vi "Day01-01.vi"() -> ()   [LabVIEW 2021]
panel:
  out "삭제된 부분":dbl[](array[numeric])
  out "부분이 삭제된 배열":dbl[](array[numeric])
  out "출력 배열":dbl[](array[numeric])
  out "원소 3":dbl
  out "원소 2":dbl
  out "원소":dbl
  out "크기 2":i32[](array[numeric])
  out "크기":i32
  in  "2D 배열":dbl[][](array[numeric])
  in  "1D 배열":dbl[](array[numeric])
  in  "배열":dbl[](array[numeric])
  in  "2차원 배열":dbl[][](array[numeric])
  in  "1차원 배열 2":dbl[](array[numeric])
  in  "1차원 배열":dbl[](array[numeric])
  in  "숫자형 11":dbl
  out "0, 1":i16
  out "결과 문자열 2":string
  out "결과 문자열":string
  out "숫자 2":i32
  out "10진수 문자열":string
  out "숫자":i32
  in  "문자열 8":string
  out "문자열 7":string
  in  "문자열 6":string
  in  "문자열 5":string
  in  "문자열 4":string
  out "길이":i32
  in  "문자열 3":string
  in  "불리언 3":bool
  out "숫자형 10":dbl
  out "32비트 정수":i32
  in  "숫자형 9":i32
  in  "숫자형 8":dbl
  in  "숫자형 7":dbl
  out "X + Y":dbl
  in  "숫자형 5":u8
  in  "숫자형 4":u8
  out "가장 가까운 정수값":dbl
  in  "숫자형 3":u32
  out "숫자형 6":dbl
  in  "Y":dbl
  in  "X":dbl
  out "불리언 2":bool
  in  "불리언":bool
  out "문자열 2":string
  in  "문자열":string
  out "숫자형 2":dbl
  in  "숫자형":dbl
  # "배열"
  # "예제 4-1"
  # "예제 4-4"
  # "원소"
  # "인덱스"
  # "예제 4-2"
  # "예제 4-5"
  # "예제 4-3"
  # "원소의 개수는? \n --> 5개"
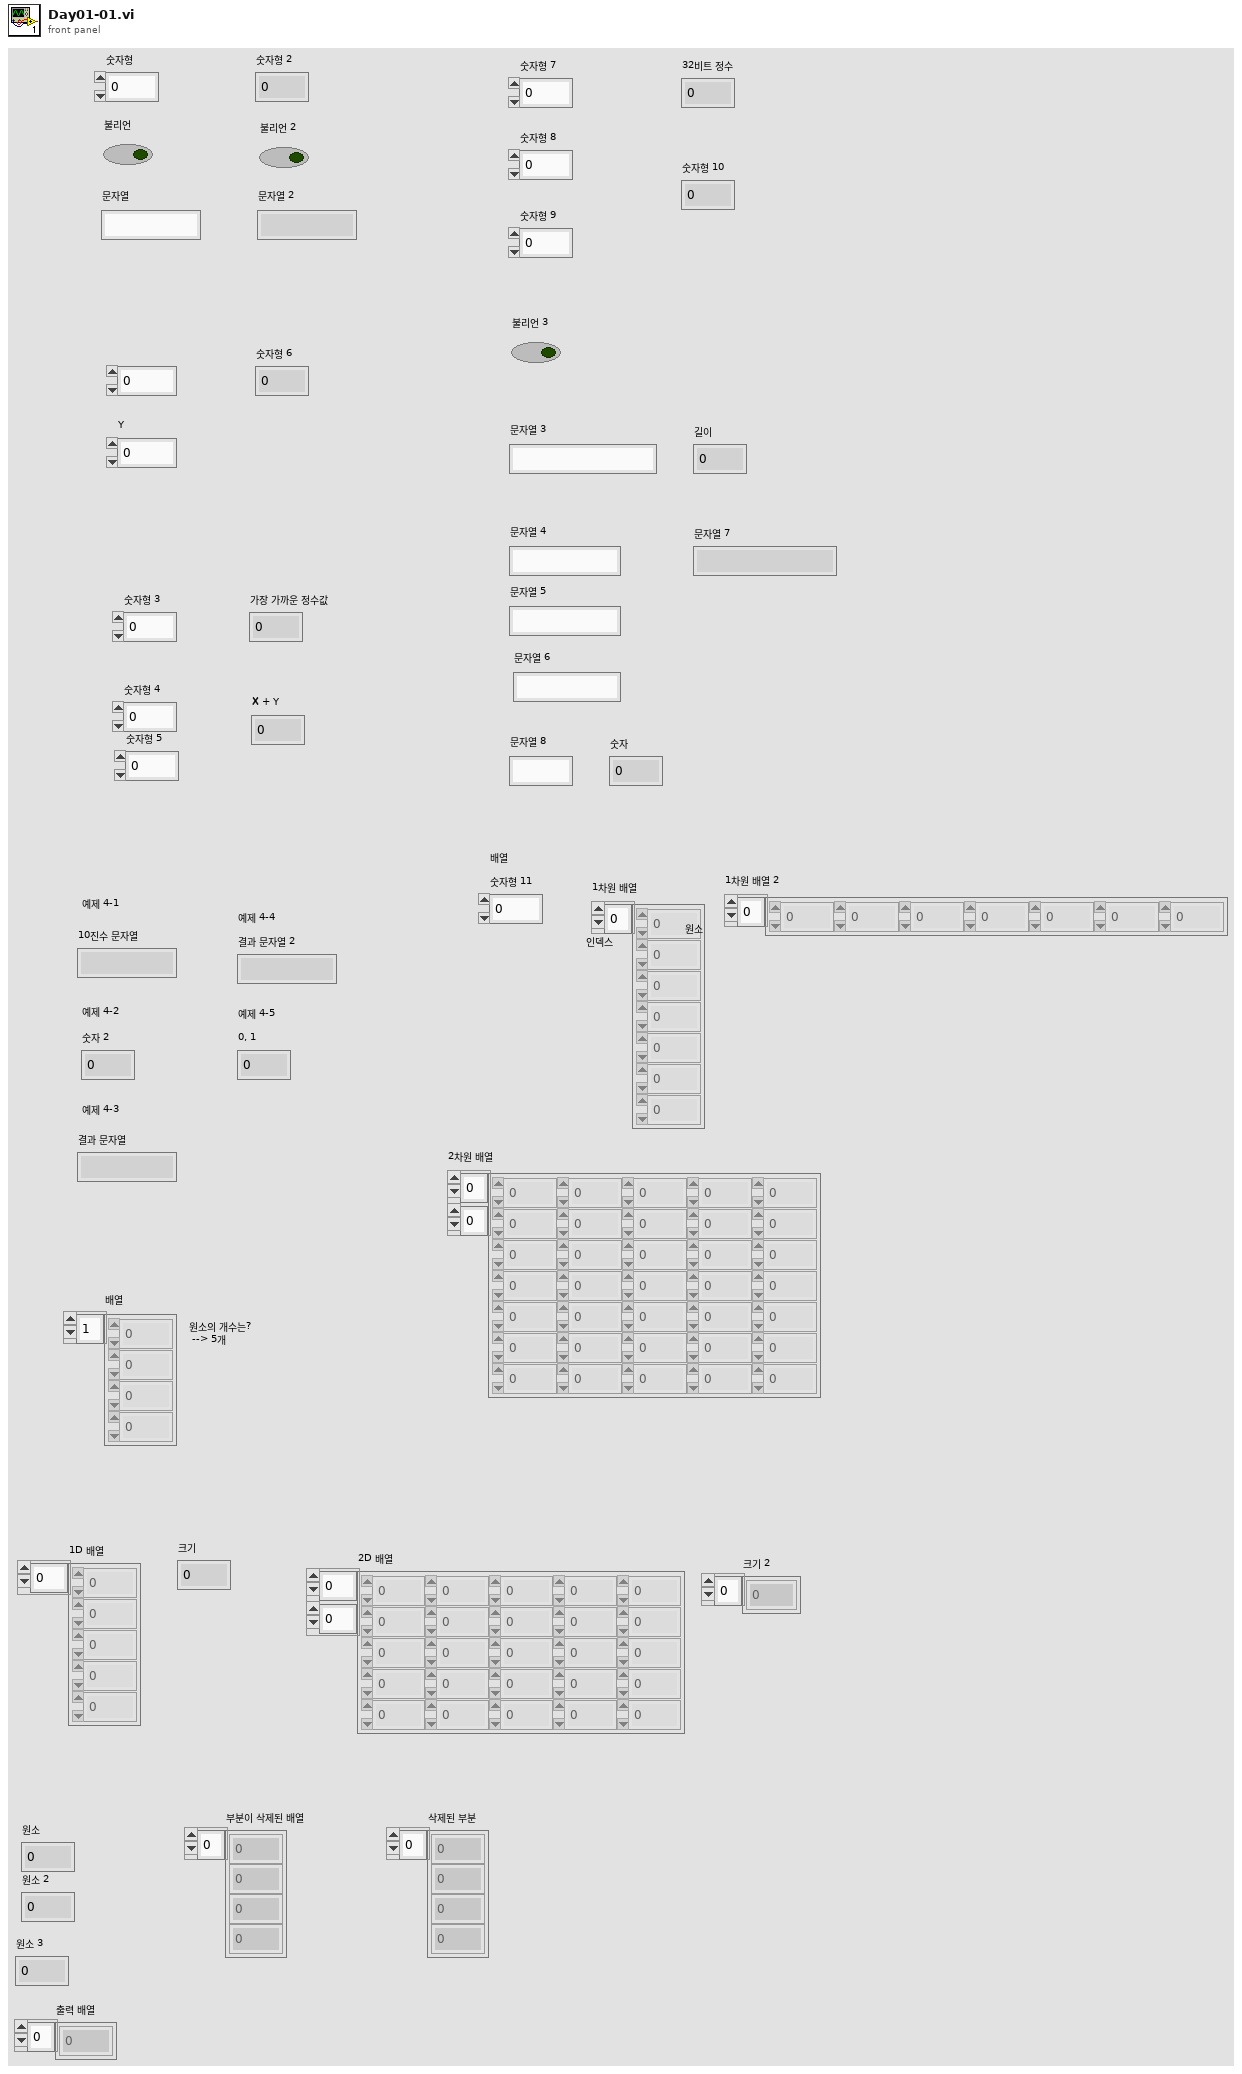
[diagram p1: front panel]
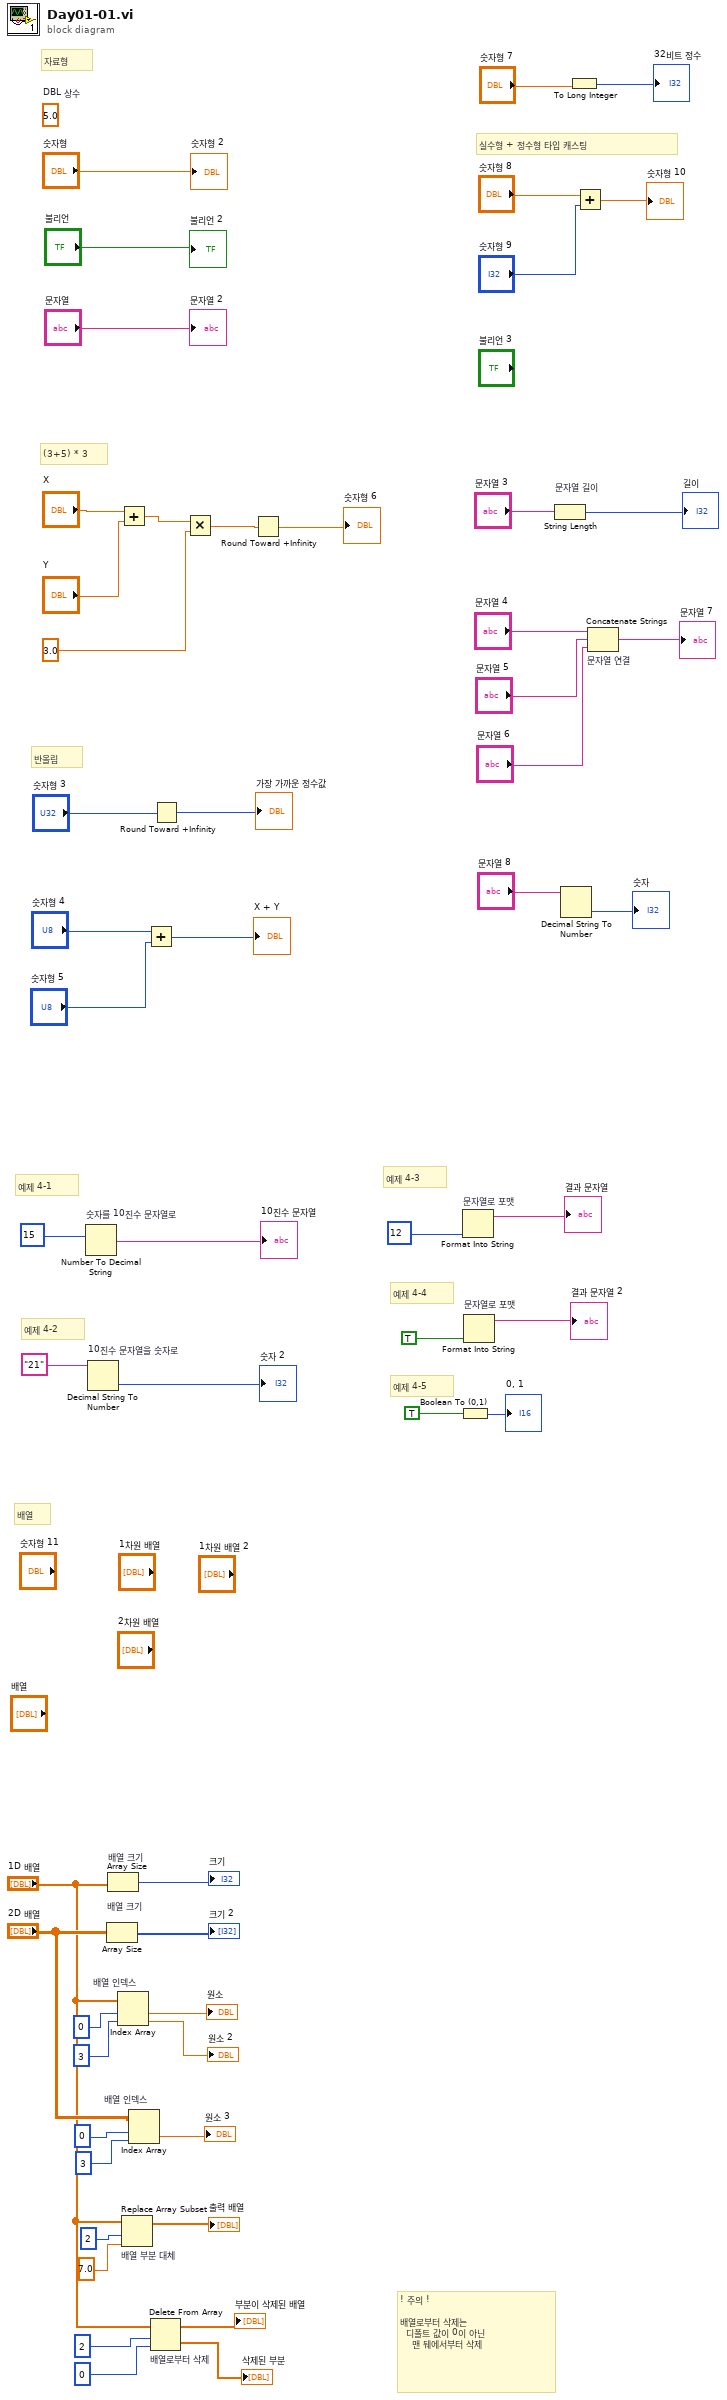
[diagram p0: block diagram]
diagram:
  (unwired) 5.0  # DBL 상수
  # "! 주의 !\n\n배열로부터 삭제는\n  디폴트 값이 0이 아닌\n    맨 뒈에서부터 삭제"
  # "배열"
  # "예제 4-5"
  # "예제 4-4"
  # "예제 4-3"
  # "예제 4-2"
  # "예제 4-1"
  # "실수형 + 정수형 타입 캐스팅"
  # "반올림"
  # "(3+5) * 3"
  # "자료형"
  n1 = Number To Decimal String "숫자를 10진수 문자열로"(number=15) -> (decimal integer string=→"10진수 문자열":string)  [unwired: 1 in]
  n2 = Decimal String To Number "10진수 문자열을 숫자로"(string="21") -> (number=→"숫자 2":i32)  [unwired: 2 in, 1 out]
  n3 = Array Size "배열 크기"(array="2D 배열") -> (size(s)=→"크기 2":i32[])
  n4 = Array Size "배열 크기"(array="1D 배열") -> (size(s)=→"크기":i32)
  n5 = Index Array "배열 인덱스"(array="1D 배열", index #1=0, index #2=3) -> (element #1=→"원소":dbl, element #2=→"원소 2":dbl)
  n6 = Add(x="X", y="Y") -> (x+y=w50:dbl)
  n7 = Replace Array Subset "배열 부분 대체"(array="1D 배열", new element=7.0 ("새 원소/부분배열"), index=2 ("인덱스")) -> (→"출력 배열":dbl[])
  n8 = Index Array "배열 인덱스"(array="2D 배열", index (row)=0, index (col)=3) -> (element=→"원소 3":dbl)
  n9 = Add(x="숫자형 4", y="숫자형 5") -> (x+y=→"X + Y":u8)
  n10 = Delete From Array "배열로부터 삭제"(array="1D 배열", length=2 ("길이"), index=0 ("인덱스")) -> (deleted portion=→"삭제된 부분":dbl[], array with subset deleted=→"부분이 삭제된 배열":dbl[])
  n11 = Round Toward +Infinity(x="숫자형 3") -> (ceil(x): smallest int >= x=→"가장 가까운 정수값":u32)
  n12 = Multiply(x=w50, y=3.0) -> (x*y=w48:dbl)
  n13 = Round Toward +Infinity(x=w48) -> (ceil(x): smallest int >= x=→"숫자형 6":dbl)
  n14 = Boolean To (0,1)(Boolean=TRUE) -> (0, 1=→"0, 1":i16)
  n15 = Format Into String "문자열로 포맷"(12) -> (resulting string=→"결과 문자열":string)  [unwired: 3 in, 1 out]
  n16 = Format Into String "문자열로 포맷"(TRUE) -> (resulting string=→"결과 문자열 2":string)  [unwired: 3 in, 1 out]
  n17 = String Length "문자열 길이"(string="문자열 3") -> (length=→"길이":i32)
  n18 = Decimal String To Number(string="문자열 8") -> (number=→"숫자":i32)  [unwired: 2 in, 1 out]
  n19 = To Long Integer(number="숫자형 7") -> (32bit integer=→"32비트 정수":i32)
  n20 = Add(x="숫자형 8", y="숫자형 9") -> (x+y=→"숫자형 10":dbl)
  n21 = Concatenate Strings "문자열 연결"("문자열 4", "문자열 5", "문자열 6") -> (→"문자열 7":string)
  "숫자형 2" <- "숫자형"
  "문자열 2" <- "문자열"
  "불리언 2" <- "불리언"
